vi "GetAllInfo.vi"(0 "reference in":refnum<class "ClassRelationshipEdge.lvclass">, 5 "error in (no error)":errorcluster) -> (14 "reference out":refnum<class "ClassRelationshipEdge.lvclass">, 16 "AllInfo":T2, 17 "PathInfo":T1, 19 "error out":errorcluster)   [LabVIEW 2012, in "ClassRelationshipEdge.lvclass"]
uses:
  <resource>/Framework/Providers/Open_GDS/UML/ClassRelationshipEdge_class/ClassRelationshipEdge.lvclass
  <resource>/Framework/Providers/Open_GDS/UML/ClassRelationshipEdge_class/GetAllInfoType.ctl
  <resource>/Framework/Providers/Open_GDS/UML/AbstractNode_class/AbstractNode.lvclass
  <resource>/Framework/Providers/Open_GDS/UML/LineStyle_class/LineStyleType.ctl
  <resource>/Framework/Providers/Open_GDS/UML/ArrowHead_class/ArrowHeadType.ctl
  <resource>/Framework/Providers/Open_GDS/UML/ClassRelationshipEdge_class/PathInfoType.ctl
  <resource>/Framework/Providers/Open_GDS/UML/BentStyle_class/BentStyle.lvclass
  <resource>/Framework/Providers/Open_GDS/UML/LineStyle_class/LineStyle.lvclass
  <resource>/Framework/Providers/Open_GDS/UML/ArrowHead_class/ArrowHead.lvclass
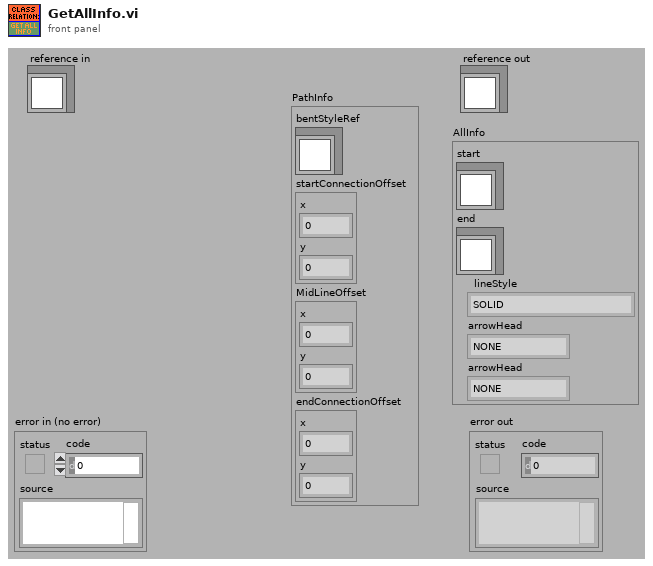
[diagram p1: front panel]
types:
  T1 = typedef "ClassRelationshipEdge.lvclass/PathInfoType.ctl" = cluster{"bentStyleRef":refnum<class "BentStyle.lvclass">, "startConnectionOffset":cluster{"x":i32, "y":i32}, "MidLineOffset":cluster{"x":i32, "y":i32}, "endConnectionOffset":cluster{"x":i32, "y":i32}}
  T2 = typedef "ClassRelationshipEdge.lvclass/GetAllInfoType.ctl" = cluster{"start":refnum<class "AbstractNode.lvclass">, "end":refnum<class "AbstractNode.lvclass">, "lineStyle":T3, "arrowHead":T4, "arrowHead":T4}
  T3 = typedef "LineStyle.lvclass/LineStyleType.ctl" = enum16{"SOLID", "DOTTED"}
  T4 = typedef "ArrowHead.lvclass/ArrowHeadType.ctl" = enum16{"NONE", "TRIANGLE", "BLACK_TRIANGLE", "V", "HALF_V", "DIAMOND", "BLACK_DIAMOND"}
  T5 = typedef "ClassRelationshipEdge.lvclass/ObjectAttributes.ctl" = cluster{"Base class":T6, "bentStyleRef":refnum<class "BentStyle.lvclass">, "startConnectionOffset":cluster{"x":i32, "y":i32}, "endConnectionOffset":cluster{"x":i32, "y":i32}, "MidLineOffset":cluster{"x":i32, "y":i32}, "DepClass":T10}
  T6 = typedef "SegmentedLineEdge.lvclass/ObjectAttributes.ctl" = cluster{"Base class":T7, "lineStyle":refnum<class "LineStyle.lvclass">, "startArrowHead":refnum<class "ArrowHead.lvclass">, "endArrowHead":refnum<class "ArrowHead.lvclass">, "startLabel":string, "midLabel":string, "endLabel":string, "MidLabelOffset":T9, "SplitWire":bool}
  T7 = typedef "GeneralPathEdge.lvclass/ObjectAttributes.ctl" = cluster{"Base class":T8}
  T8 = typedef "AbstractEdge.lvclass/ObjectAttributes.ctl" = cluster{"start":refnum<class "AbstractNode.lvclass">, "end":refnum<class "AbstractNode.lvclass">}
  T9 = typedef "Point Point2D.ctl" = cluster{"x":dbl, "y":dbl}
  T10 = typedef "ReversedEngineering_ViDependencyDetailsType.ctl" = cluster{"ThisVIs/Ctls":path[], "Dependent_VIs/Ctls":path[]}
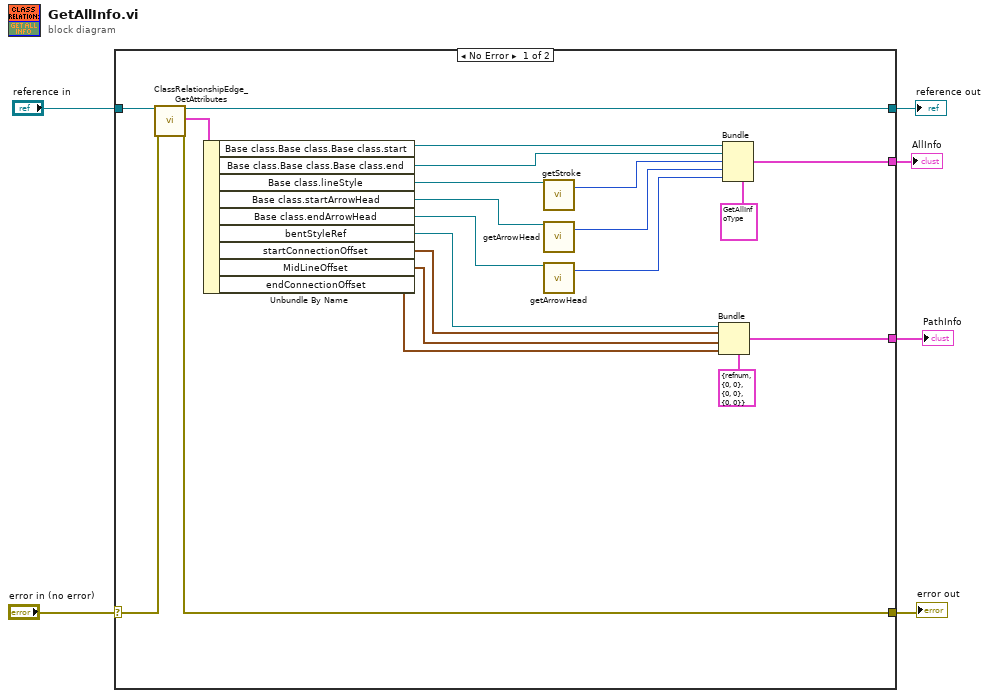
[diagram p0: block diagram]
diagram:
  n1 = case shown="No Error" "error in (no error)" {
    selector: "error in (no error)" -> [w27 w29]
    tunnel: [w25 w29] -> w5
    tunnel: [w23 w28] -> w3
    tunnel: "reference in" -> [w24 w28]
    tunnel: [w13 _] -> w2
    tunnel: [w10 _] -> w1
    frame No Error {
      n2 = call <resource>:"ClassRelationshipEdge_GetAttributes.vi"("reference in"=w24, "error in (no error)"=w27) -> ("reference out"=w23:refnum<class "ClassRelationshipEdge.lvclass">, "Attributes"=w26:T5, "error out"=w25:errorcluster)  [unwired: 14 in, 1 out]
      n3 = Unbundle By Name(w26) -> ("Base class.Base class.Base class.start"=w21:refnum<class "AbstractNode.lvclass">, "Base class.Base class.Base class.end"=w20:refnum<class "AbstractNode.lvclass">, "Base class.lineStyle"=w22:refnum<class "LineStyle.lvclass">, "Base class.startArrowHead"=w18:refnum<class "ArrowHead.lvclass">, "Base class.endArrowHead"=w16:refnum<class "ArrowHead.lvclass">, "bentStyleRef"=w12:refnum<class "BentStyle.lvclass">, "startConnectionOffset"=w11:cluster{"x":i32, "y":i32}, "MidLineOffset"=w9:cluster{"x":i32, "y":i32}, "endConnectionOffset"=w8:cluster{"x":i32, "y":i32})
      n4 = call-dynamic "getStroke.vi"("reference"=w22) -> ("lineStyle"=w19:T3)  [unwired: 16 in, 2 out]
      n5 = call <resource>:"getArrowHead.vi"("reference"=w18) -> ("arrowHead"=w17:T4)  [unwired: 16 in, 2 out]
      n6 = call <resource>:"getArrowHead.vi"("reference"=w16) -> ("arrowHead"=w15:T4)  [unwired: 16 in, 2 out]
      n7 = Bundle(cluster=T1 {"bentStyleRef"=refnum, "startConnectionOffset"={"x"=0, "y"=0}, "MidLineOffset"={"x"=0, "y"=0}, "endConnectionOffset"={"x"=0, "y"=0}} ("PathInfo"), "bentStyleRef"=w12, "startConnectionOffset"=w11, "MidLineOffset"=w9, "endConnectionOffset"=w8) -> (w10:T1)
      n8 = Bundle(cluster=T2 {"start"=refnum, "end"=refnum, "lineStyle"=enum."SOLID", "arrowHead"=enum."NONE", "arrowHead"=enum."NONE"} ("output cluster"), "start"=w21, "end"=w20, "lineStyle"=w19, "arrowHead"=w17, "arrowHead"=w15) -> (w13:T2)
    }
    frame Error {
    }
  }
  "error out" <- w5
  "reference out" <- w3
  "AllInfo" <- w2
  "PathInfo" <- w1
